vi "shooter_flywheel.vi"(8 "Low goal RPM":dbl=1500.0, 9 "High goal RPM":dbl=4000.0, 10 "Flywheel":bool, 11 "High goal?":bool) -> (2 "Flywheel RPM":cluster{"RPM":dbl, "Flywheel Setpoint RPM":dbl}(graph), 5 "error from goal":dbl, 7 "Closed-loop Error":dbl format="%.2f")   [LabVIEW 2020]
uses:
  <vilib>/Rock Robotics/WPI/ThirdParty/Phoenix-LabVIEW/Motor Controller/Controls/CTRE_Phoenix_MotorControl_ControlMode.ctl
  <vilib>/Rock Robotics/WPI/ThirdParty/JAS_Junk/TrajLib/SimpleMotorFF_Calculate.vi
  TitanLib/Lib/RPMToRawUnits-2048-CPR.vi
  <vilib>/Rock Robotics/WPI/ThirdParty/Phoenix-LabVIEW/Motor Controller/Get/CTRE_Phoenix_MotorController_GetSelectedSensorData.vi
  TitanLib/Lib/RawUnitsToRPM-2048-CPR.vi
  <vilib>/Rock Robotics/Network Tables/NT Write Number.vi
  <vilib>/Rock Robotics/WPI/ThirdParty/Phoenix-LabVIEW/Motor Controller/Get/CTRE_Phoenix_MotorController_GetVoltage.vi
  TitanLib/Lib/TitanLib.lvlib
  <vilib>/Rock Robotics/WPI/ThirdParty/JAS_Junk/TrajLib/Trajectory_Library.lvlib
panel:
  in  "Tolerance":dbl
  in  "kA":dbl
  out "Output Voltage":dbl(graph)
  in  "Flywheel PIDF":T1={"Set Constants"=FALSE, "P"=0.00029748, "I"=0.0, "D"=0.0, "F"=0.0, "I Zone"=0.0, "Cruise Velocity"=0, "Acceleration"=0, "Percent Deadband"=0.0}
  in  "kV":dbl=0.114
  in  "kS":dbl=0.1309
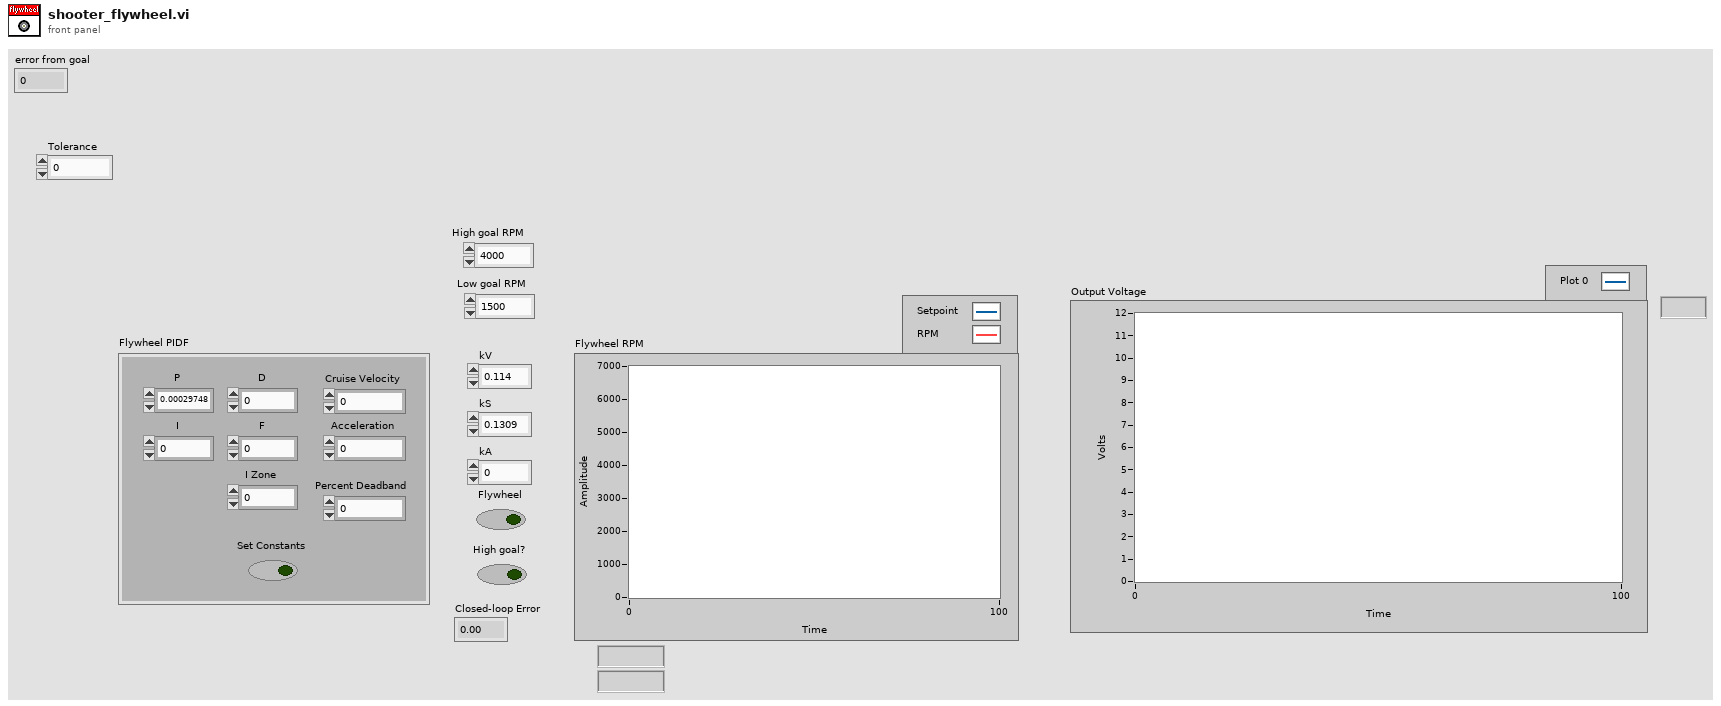
[diagram p1: front panel]
types:
  T1 = cluster{"Set Constants":bool, "P":dbl, "I":dbl, "D":dbl, "F":dbl, "I Zone":dbl, "Cruise Velocity":i32, "Acceleration":i32, "Percent Deadband":dbl}
  T2 = typedef "Trajectory_Library.lvlib/SIMPLE_MOTOR_FF.ctl" = cluster{"Ks":dbl, "Kv":dbl, "Ka":dbl}
  T3 = typedef "WPI_MotorControlDeviceRef.ctl" = cluster{"DeviceStatus":errorcluster, "Type":T4, "PWM":cluster{"PWM Channel":T5, "DeadBand":T6}, "CAN":cluster{"Device Number":u8, "SetOutput VI Ref":variant, "GetOutput VI Ref":variant, "Enable VI Ref":variant, "Disable VI Ref":variant, "Data":variant}, "Invert":bool, "DIO PWM":cluster{"PWM \"Enable\" Channel":T5, "DIOChannel":T7, "PWM Rate":dbl}}
  T4 = typedef "WPI_MotorControlType.ctl" = enum16{"PWM", "CAN", "DIO PWM"}
  T5 = typedef "FPGA_DIOPWMChannel.ctl" = enum8{"PWM 0", "PWM 1", "PWM 2", "PWM 3", "PWM 4", "PWM 5", "PWM 6", "PWM 7", "PWM 8", "PWM 9", "PWM MXP 0", "PWM MXP 1", "PWM MXP 2", "PWM MXP 3", "PWM MXP 4", "PWM MXP 5", "PWM MXP 6", "PWM MXP 7", "PWM MXP 8", "PWM MXP 9", "Invalid"}
  T6 = typedef "WPI_PWMDeadband.ctl" = cluster{"Name":string, "maxPositivePwm":i32, "minPositivePwm":i32, "centerPwm":i32, "maxNegativePwm":i32, "minNegativePwm":i32, "angularRange":u16}
  T7 = typedef "FPGA_DIOChannel.ctl" = enum8{"DIO 0", "DIO 1", "DIO 2", "DIO 3", "DIO 4", "DIO 5", "DIO 6", "DIO 7", "DIO 8", "DIO 9", "DIO MXP 0", "DIO MXP 1", "DIO MXP 2", "DIO MXP 3", "DIO MXP 4", "DIO MXP 5", "DIO MXP 6", "DIO MXP 7", "DIO MXP 8", "DIO MXP 9", "DIO MXP 10", "DIO MXP 11", "DIO MXP 12", "DIO MXP 13", "DIO MXP 14", "DIO MXP 15", "SPI Port CS1", "SPI Port CS2", "SPI Port CS3", "SPI Port MISO", "SPI Port MOSI", "Invalid"}
  T8 = typedef "CTRE_Phoenix_MotorControl_ControlMode.ctl" = u16
  T9 = enum16{"DemandType_Neutral", "DemandType_AuxPID", "DemandType_ArbitraryFeedForward"}
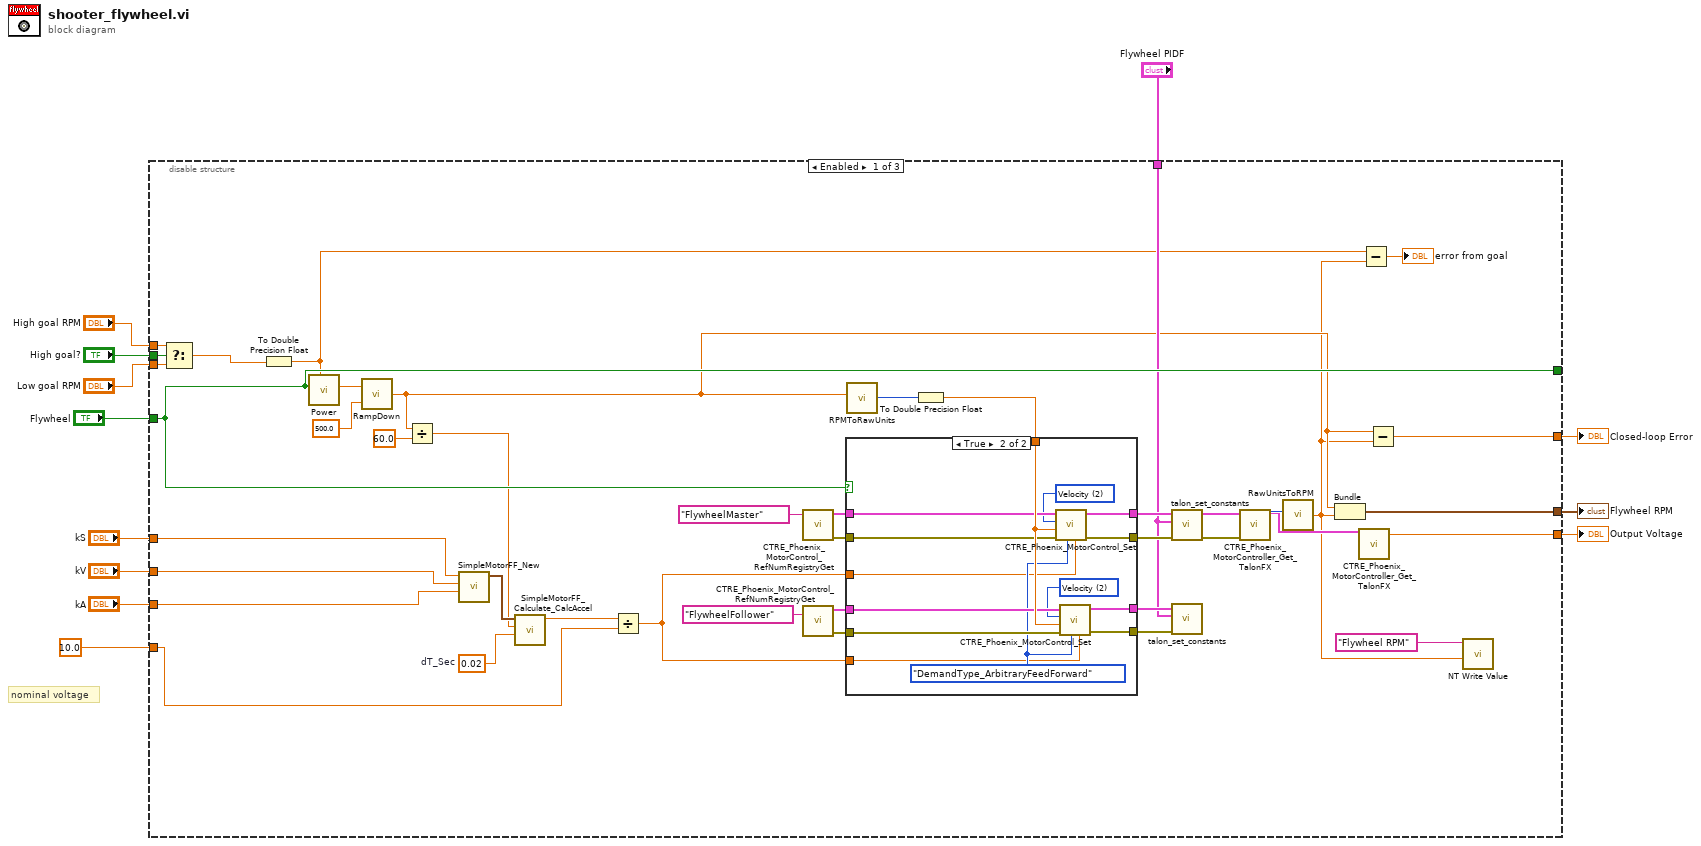
[diagram p0: block diagram]
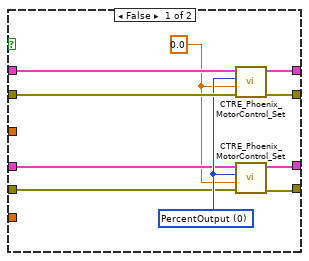
[diagram p2: hidden frame]
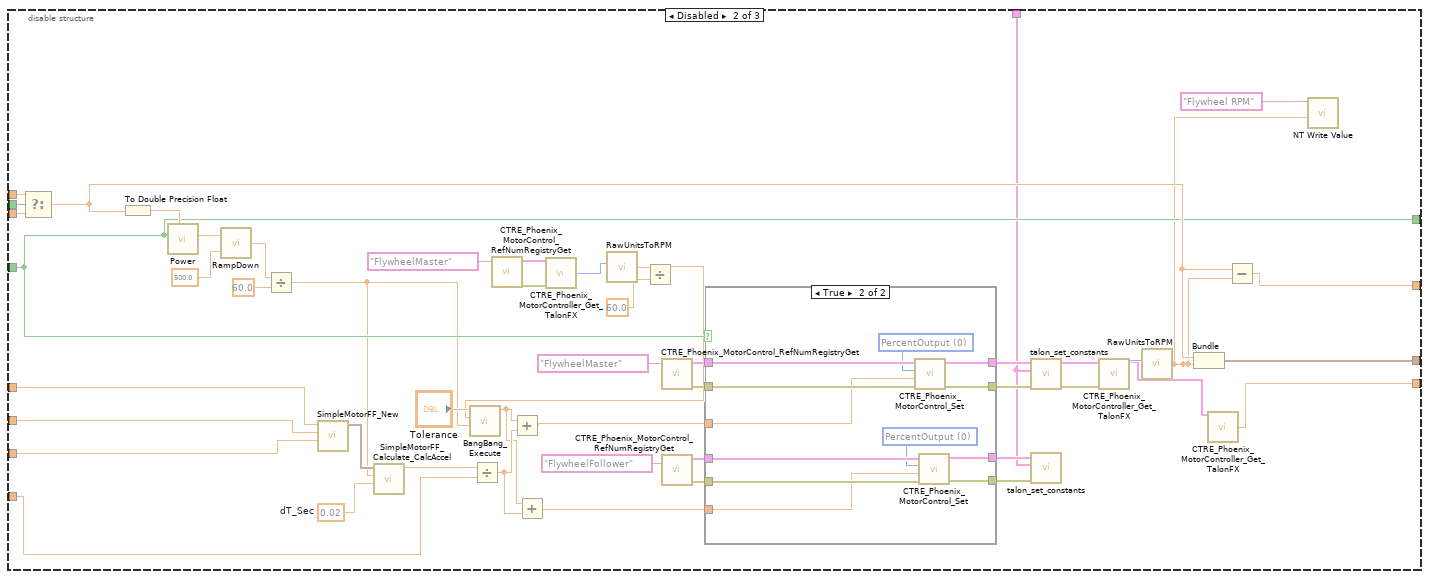
[diagram p3: hidden frame]
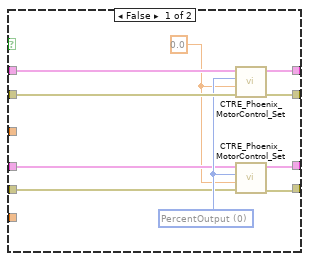
[diagram p4: hidden frame]
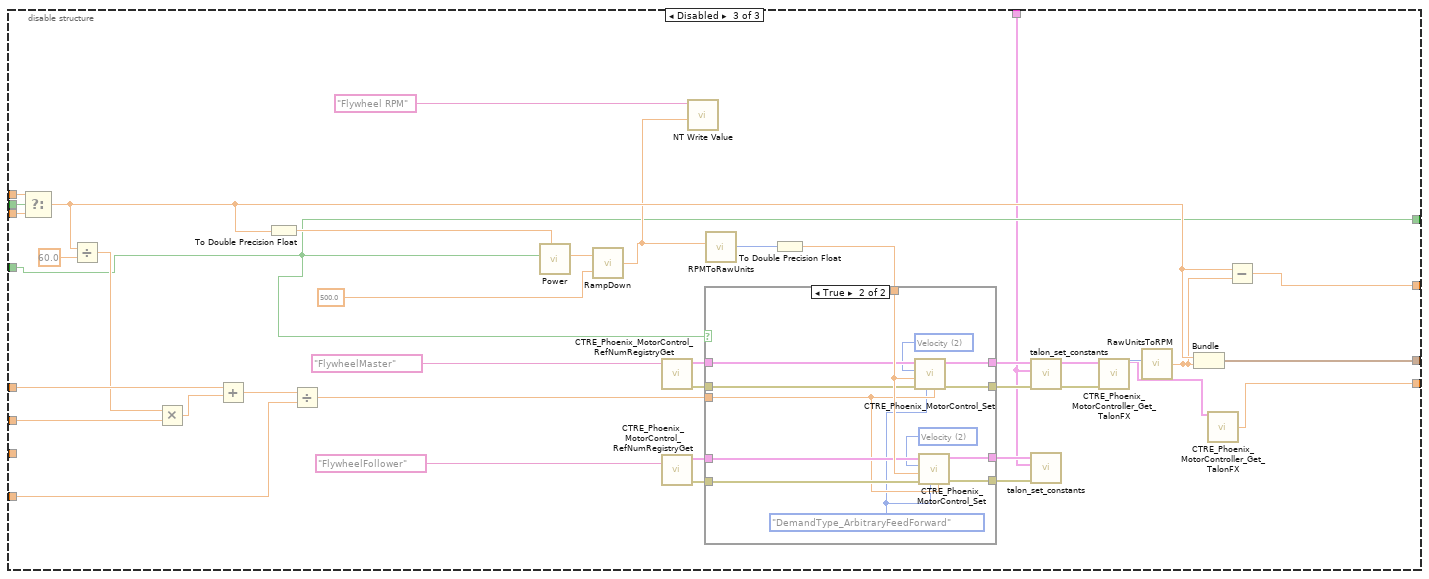
[diagram p5: hidden frame]
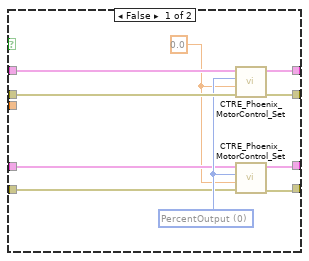
[diagram p6: hidden frame]
diagram:
  # "nominal voltage"
  n1 = disable-structure shown="Enabled" {
    disable-tunnel: 10.0 ("y") -> [w20 w94 w184]
    disable-tunnel: "kS" -> [w22 w95 w181]
    disable-tunnel: "kV" -> [w23 w96 w180]
    disable-tunnel: "High goal?" -> [w37 w112 w163]
    disable-tunnel: "Low goal RPM" -> [w36 w111 w162]
    disable-tunnel: "High goal RPM" -> [w35 w110 w161]
    disable-tunnel: [w34 w109 w160] -> w4
    disable-tunnel: [w31 w105 w154] -> _
    disable-tunnel: "Flywheel" -> [w31 w105 w154]
    disable-tunnel: "Flywheel PIDF" -> [w30 w104 w153]
    disable-tunnel: [w29 w103 w152] -> w3
    disable-tunnel: [w28 w102 w151] -> w2
    disable-tunnel: "kA" -> [w24 w97 _]
    frame Enabled {
      w26 = 0.02  # dT_Sec
      n2 = Select(t=w35, s=w37, f=w36) -> (s? t:f=w17:dbl)
      n3 = To Double Precision Float(number=w17) -> (double precision float=w15:dbl)
      n4 = call "Power.vi"("Positive Power"=w15, "Positive"=w31) -> ("Output"=w49:dbl)  [unwired: 9 in]
      n5 = call "RampDown.vi"("Decrease per Cycle"=500.0, "Input"=w49) -> ("Output"=w16:dbl)
      n6 = Divide(x=w16, y=60.0) -> (x/y=w21:dbl)
      n7 = call <vilib>:"SimpleMotorFF_New.vi"("Ka"=w24, "Kv"=w23, "Ks"=w22) -> ("SIMPLE_MOTOR_FF"=w25:T2)  [unwired: 8 in]
      n8 = call <vilib>:"SimpleMotorFF_Calculate_CalcAccel.vi"("dT_Sec"=w26, "Vel"=w21, "SIMPLE_MOTOR_FF"=w25) -> ("FeedForward"=w19:dbl)  [unwired: 8 in]
      n9 = Divide(x=w19, y=w20) -> (x/y=w18:dbl)
      n10 = call <vilib>:"CTRE_Phoenix_MotorControl_RefNumRegistryGet.vi"("refnum name"="FlywheelMaster") -> ("error out"=w46:errorcluster, "PhoenixMotorControlDevRef"=w45:T3)  [unwired: 9 in]
      n11 = call <vilib>:"CTRE_Phoenix_MotorControl_RefNumRegistryGet.vi"("refnum name"="FlywheelFollower") -> ("error out"=w48:errorcluster, "PhoenixMotorControlDevRef"=w47:T3)  [unwired: 9 in]
      n12 = call-poly "RPMToRawUnits.vi"("RPM"=w16) -> ("Raw Units"=w41:i32)  [unwired: 3 in]
      n13 = To Double Precision Float(number=w41) -> (double precision float=w40:dbl)
      n14 = case shown="True" w31 {
        tunnel: [w58 w78] -> w54
        tunnel: [w59 w77] -> w53
        tunnel: [w57 w76] -> w52
        tunnel: [w56 w75] -> w51
        tunnel: w40 -> [_ w74]
        tunnel: w48 -> [w60 w73]
        tunnel: w47 -> [w61 w72]
        tunnel: w46 -> [w64 w70]
        tunnel: w45 -> [w63 w69]
        tunnel: w18 -> [_ w66]
        tunnel: w18 -> [_ w65]
        frame False {
          w55 = 0.0 ("Output")
          w62 = T8 0 items=["PercentOutput"=0, "Position"=1, "Velocity"=2, "Current"=3, "Follower"=5, "MotionProfile"=6, "MotionMagic"=7, "MotionProfileArc"=10, "Disabled"=15] ("Control Mode")
          n15 = call <vilib>:"CTRE_Phoenix_MotorControl_Set.vi"("error in (no error)"=w64, "Output"=w55, "Control Mode"=w62, "PhoenixMotorControlDevRef"=w63) -> ("error out"=w57:errorcluster, "PhoenixMotorControlDevRef"=w56:T3)  [unwired: 6 in]
          n16 = call <vilib>:"CTRE_Phoenix_MotorControl_Set.vi"("error in (no error)"=w60, "Output"=w55, "Control Mode"=w62, "PhoenixMotorControlDevRef"=w61) -> ("error out"=w58:errorcluster, "PhoenixMotorControlDevRef"=w59:T3)  [unwired: 6 in]
        }
        frame True {
          w67 = T9."DemandType_ArbitraryFeedForward" ("DemandType")
          w71 = T8 2 items=["PercentOutput"=0, "Position"=1, "Velocity"=2, "Current"=3, "Follower"=5, "MotionProfile"=6, "MotionMagic"=7, "MotionProfileArc"=10, "Disabled"=15] ("Control Mode")
          w68 = T8 2 items=["PercentOutput"=0, "Position"=1, "Velocity"=2, "Current"=3, "Follower"=5, "MotionProfile"=6, "MotionMagic"=7, "MotionProfileArc"=10, "Disabled"=15] ("Control Mode")
          n17 = call <vilib>:"CTRE_Phoenix_MotorControl_Set.vi"("Demand1"=w65, "DemandType"=w67, "error in (no error)"=w70, "Output"=w74, "Control Mode"=w68, "PhoenixMotorControlDevRef"=w69) -> ("error out"=w76:errorcluster, "PhoenixMotorControlDevRef"=w75:T3)  [unwired: 4 in]
          n18 = call <vilib>:"CTRE_Phoenix_MotorControl_Set.vi"("Demand1"=w66, "DemandType"=w67, "error in (no error)"=w73, "Output"=w74, "Control Mode"=w71, "PhoenixMotorControlDevRef"=w72) -> ("error out"=w78:errorcluster, "PhoenixMotorControlDevRef"=w77:T3)  [unwired: 4 in]
        }
      }
      n19 = call "talon_set_constants.vi"("error in"=w52, "Constants"=w30, "PhoenixMotorControlDevRef"=w51) -> ("error out"=w38:errorcluster, "PhoenixMotorControlDevRef"=w39:T3)  [unwired: 7 in]
      n20 = call "talon_set_constants.vi"("error in"=w54, "Constants"=w30, "PhoenixMotorControlDevRef"=w53) -> ()  [unwired: 7 in, 2 out]
      n21 = call-poly <vilib>:"CTRE_Phoenix_MotorController_Get_TalonFX.vi"("PhoenixMotorControlDevRef"=w39, "error in"=w38) -> ("PhoenixMotorControlDevRef"=w33:T3, "Velocity (Raw Sensor Units per 100 ms)"=w42:i32)  [unwired: 10 in, 2 out]
      n22 = call-poly "RawUnitsToRPM.vi"("Raw Units"=w42) -> ("RPM"=w14:dbl)  [unwired: 3 in]
      n23 = Bundle("Output"=w16, "RPM"=w14) -> (w29:cluster{"Output":dbl, "RPM":dbl})  [unwired: 1 in]
      n24 = call-poly <vilib>:"CTRE_Phoenix_MotorController_Get_TalonFX.vi"("PhoenixMotorControlDevRef"=w33) -> ("Output Voltage"=w34:dbl)  [unwired: 10 in, 4 out]
      n25 = Subtract(x=w15, y=w14) -> (x-y=→"error from goal":dbl)
      n26 = Subtract(x=w16, y=w14) -> (x-y=w28:dbl)
      n27 = call-poly <vilib>:"NT Write Value.vi"("Numeric"=w14, "Name"="Flywheel RPM") -> ()  [unwired: 9 in, 1 out]
    }
    frame Disabled {
      w99 = 0.02  # dT_Sec
      n28 = Select(t=w110, s=w112, f=w111) -> (s? t:f=w107:dbl)
      n29 = To Double Precision Float(number=w107) -> (double precision float=w116:dbl)
      n30 = call "Power.vi"("Positive Power"=w116, "Positive"=w105) -> ("Output"=w123:dbl)  [unwired: 9 in]
      n31 = call "RampDown.vi"("Decrease per Cycle"=500.0, "Input"=w123) -> ("Output"=w101:dbl)
      n32 = Divide(x=w101, y=60.0) -> (x/y=w82:dbl)
      n33 = call <vilib>:"SimpleMotorFF_New.vi"("Ka"=w97, "Kv"=w96, "Ks"=w95) -> ("SIMPLE_MOTOR_FF"=w98:T2)  [unwired: 8 in]
      n34 = call <vilib>:"SimpleMotorFF_Calculate_CalcAccel.vi"("dT_Sec"=w99, "Vel"=w82, "SIMPLE_MOTOR_FF"=w98) -> ("FeedForward"=w93:dbl)  [unwired: 8 in]
      n35 = Divide(x=w93, y=w94) -> (x/y=w84:dbl)
      n36 = call <vilib>:"CTRE_Phoenix_MotorControl_RefNumRegistryGet.vi"("refnum name"="FlywheelMaster") -> ("error out"=w79:errorcluster, "PhoenixMotorControlDevRef"=w80:T3)  [unwired: 9 in]
      n37 = call-poly <vilib>:"CTRE_Phoenix_MotorController_Get_TalonFX.vi"("PhoenixMotorControlDevRef"=w80, "error in"=w79) -> ("Velocity (Raw Sensor Units per 100 ms)"=w86:i32)  [unwired: 10 in, 3 out]
      n38 = call-poly "RawUnitsToRPM.vi"("Raw Units"=w86) -> ("RPM"=w87:dbl)  [unwired: 3 in]
      n39 = Divide(x=w87, y=60.0) -> (x/y=w83:dbl)
      n40 = call <vilib>:"BangBang_Execute.vi"("Setpoint"=w82, "Measurment"=w83, "Tolerance"="Tolerance") -> ("ControlOutput"=w81:dbl)  [unwired: 6 in, 2 out]
      n41 = Add(x=w81, y=w84) -> (x+y=w91:dbl)
      n42 = Add(x=w81, y=w84) -> (x+y=w90:dbl)
      n43 = call <vilib>:"CTRE_Phoenix_MotorControl_RefNumRegistryGet.vi"("refnum name"="FlywheelMaster") -> ("error out"=w120:errorcluster, "PhoenixMotorControlDevRef"=w119:T3)  [unwired: 9 in]
      n44 = call <vilib>:"CTRE_Phoenix_MotorControl_RefNumRegistryGet.vi"("refnum name"="FlywheelFollower") -> ("error out"=w122:errorcluster, "PhoenixMotorControlDevRef"=w121:T3)  [unwired: 9 in]
      n45 = case shown="True" w105 {
        tunnel: [w132 w150] -> w128
        tunnel: [w133 w149] -> w127
        tunnel: [w131 w148] -> w126
        tunnel: [w130 w147] -> w125
        tunnel: w122 -> [w134 w146]
        tunnel: w121 -> [w135 w145]
        tunnel: w120 -> [w138 w143]
        tunnel: w119 -> [w137 w142]
        tunnel: w90 -> [_ w139]
        tunnel: w91 -> [_ w140]
        frame False {
          w129 = 0.0 ("Output")
          w136 = T8 0 items=["PercentOutput"=0, "Position"=1, "Velocity"=2, "Current"=3, "Follower"=5, "MotionProfile"=6, "MotionMagic"=7, "MotionProfileArc"=10, "Disabled"=15] ("Control Mode")
          n46 = call <vilib>:"CTRE_Phoenix_MotorControl_Set.vi"("error in (no error)"=w138, "Output"=w129, "Control Mode"=w136, "PhoenixMotorControlDevRef"=w137) -> ("error out"=w131:errorcluster, "PhoenixMotorControlDevRef"=w130:T3)  [unwired: 6 in]
          n47 = call <vilib>:"CTRE_Phoenix_MotorControl_Set.vi"("error in (no error)"=w134, "Output"=w129, "Control Mode"=w136, "PhoenixMotorControlDevRef"=w135) -> ("error out"=w132:errorcluster, "PhoenixMotorControlDevRef"=w133:T3)  [unwired: 6 in]
        }
        frame True {
          w144 = T8 0 items=["PercentOutput"=0, "Position"=1, "Velocity"=2, "Current"=3, "Follower"=5, "MotionProfile"=6, "MotionMagic"=7, "MotionProfileArc"=10, "Disabled"=15] ("Control Mode")
          w141 = T8 0 items=["PercentOutput"=0, "Position"=1, "Velocity"=2, "Current"=3, "Follower"=5, "MotionProfile"=6, "MotionMagic"=7, "MotionProfileArc"=10, "Disabled"=15] ("Control Mode")
          n48 = call <vilib>:"CTRE_Phoenix_MotorControl_Set.vi"("error in (no error)"=w143, "Output"=w140, "Control Mode"=w141, "PhoenixMotorControlDevRef"=w142) -> ("error out"=w148:errorcluster, "PhoenixMotorControlDevRef"=w147:T3)  [unwired: 6 in]
          n49 = call <vilib>:"CTRE_Phoenix_MotorControl_Set.vi"("error in (no error)"=w146, "Output"=w139, "Control Mode"=w144, "PhoenixMotorControlDevRef"=w145) -> ("error out"=w150:errorcluster, "PhoenixMotorControlDevRef"=w149:T3)  [unwired: 6 in]
        }
      }
      n50 = call "talon_set_constants.vi"("error in"=w126, "Constants"=w104, "PhoenixMotorControlDevRef"=w125) -> ("error out"=w113:errorcluster, "PhoenixMotorControlDevRef"=w114:T3)  [unwired: 7 in]
      n51 = call "talon_set_constants.vi"("error in"=w128, "Constants"=w104, "PhoenixMotorControlDevRef"=w127) -> ()  [unwired: 7 in, 2 out]
      n52 = call-poly <vilib>:"CTRE_Phoenix_MotorController_Get_TalonFX.vi"("PhoenixMotorControlDevRef"=w114, "error in"=w113) -> ("PhoenixMotorControlDevRef"=w108:T3, "Velocity (Raw Sensor Units per 100 ms)"=w115:i32)  [unwired: 10 in, 2 out]
      n53 = call-poly "RawUnitsToRPM.vi"("Raw Units"=w115) -> ("RPM"=w92:dbl)  [unwired: 3 in]
      n54 = Bundle("Low goal RPM"=w107, "RPM"=w92) -> (w103:cluster{"Low goal RPM":dbl, "RPM":dbl})  [unwired: 1 in]
      n55 = call-poly <vilib>:"CTRE_Phoenix_MotorController_Get_TalonFX.vi"("PhoenixMotorControlDevRef"=w108) -> ("Output Voltage"=w109:dbl)  [unwired: 10 in, 4 out]
      n56 = Subtract(x=w107, y=w92) -> (x-y=w102:dbl)
      n57 = call-poly <vilib>:"NT Write Value.vi"("Numeric"=w92, "Name"="Flywheel RPM") -> ()  [unwired: 9 in, 1 out]
    }
    frame Disabled {
      n58 = Select(t=w161, s=w163, f=w162) -> (s? t:f=w158:dbl)
      n59 = Divide(x=w158, y=60.0) -> (x/y=w169:dbl)
      n60 = Multiply(x=w169, y=w180) -> (x*y=w182:dbl)
      n61 = Add(x=w181, y=w182) -> (x+y=w183:dbl)
      n62 = To Double Precision Float(number=w158) -> (double precision float=w171:dbl)
      n63 = Divide(x=w183, y=w184) -> (x/y=w185:dbl)
      n64 = call "Power.vi"("Positive Power"=w171, "Positive"=w154) -> ("Output"=w178:dbl)  [unwired: 9 in]
      n65 = call "RampDown.vi"("Decrease per Cycle"=500.0, "Input"=w178) -> ("Output"=w155:dbl)
      n66 = call <vilib>:"CTRE_Phoenix_MotorControl_RefNumRegistryGet.vi"("refnum name"="FlywheelMaster") -> ("error out"=w175:errorcluster, "PhoenixMotorControlDevRef"=w174:T3)  [unwired: 9 in]
      n67 = call <vilib>:"CTRE_Phoenix_MotorControl_RefNumRegistryGet.vi"("refnum name"="FlywheelFollower") -> ("error out"=w177:errorcluster, "PhoenixMotorControlDevRef"=w176:T3)  [unwired: 9 in]
      n68 = call-poly <vilib>:"NT Write Value.vi"("Numeric"=w155, "Name"="Flywheel RPM") -> ()  [unwired: 9 in, 1 out]
      n69 = call-poly "RPMToRawUnits.vi"("RPM"=w155) -> ("Raw Units"=w167:i32)  [unwired: 3 in]
      n70 = To Double Precision Float(number=w167) -> (double precision float=w166:dbl)
      n71 = case shown="True" w154 {
        tunnel: [w193 w212] -> w189
        tunnel: [w194 w211] -> w188
        tunnel: [w192 w210] -> w187
        tunnel: [w191 w209] -> w186
        tunnel: w185 -> [_ w201]
        tunnel: w166 -> [_ w208]
        tunnel: w177 -> [w195 w207]
        tunnel: w176 -> [w196 w206]
        tunnel: w175 -> [w199 w204]
        tunnel: w174 -> [w198 w203]
        frame False {
          w190 = 0.0 ("Output")
          w197 = T8 0 items=["PercentOutput"=0, "Position"=1, "Velocity"=2, "Current"=3, "Follower"=5, "MotionProfile"=6, "MotionMagic"=7, "MotionProfileArc"=10, "Disabled"=15] ("Control Mode")
          n72 = call <vilib>:"CTRE_Phoenix_MotorControl_Set.vi"("error in (no error)"=w199, "Output"=w190, "Control Mode"=w197, "PhoenixMotorControlDevRef"=w198) -> ("error out"=w192:errorcluster, "PhoenixMotorControlDevRef"=w191:T3)  [unwired: 6 in]
          n73 = call <vilib>:"CTRE_Phoenix_MotorControl_Set.vi"("error in (no error)"=w195, "Output"=w190, "Control Mode"=w197, "PhoenixMotorControlDevRef"=w196) -> ("error out"=w193:errorcluster, "PhoenixMotorControlDevRef"=w194:T3)  [unwired: 6 in]
        }
        frame True {
          w200 = T9."DemandType_ArbitraryFeedForward" ("DemandType")
          w205 = T8 2 items=["PercentOutput"=0, "Position"=1, "Velocity"=2, "Current"=3, "Follower"=5, "MotionProfile"=6, "MotionMagic"=7, "MotionProfileArc"=10, "Disabled"=15] ("Control Mode")
          w202 = T8 2 items=["PercentOutput"=0, "Position"=1, "Velocity"=2, "Current"=3, "Follower"=5, "MotionProfile"=6, "MotionMagic"=7, "MotionProfileArc"=10, "Disabled"=15] ("Control Mode")
          n74 = call <vilib>:"CTRE_Phoenix_MotorControl_Set.vi"("Demand1"=w201, "DemandType"=w200, "error in (no error)"=w204, "Output"=w208, "Control Mode"=w202, "PhoenixMotorControlDevRef"=w203) -> ("error out"=w210:errorcluster, "PhoenixMotorControlDevRef"=w209:T3)  [unwired: 4 in]
          n75 = call <vilib>:"CTRE_Phoenix_MotorControl_Set.vi"("Demand1"=w201, "DemandType"=w200, "error in (no error)"=w207, "Output"=w208, "Control Mode"=w205, "PhoenixMotorControlDevRef"=w206) -> ("error out"=w212:errorcluster, "PhoenixMotorControlDevRef"=w211:T3)  [unwired: 4 in]
        }
      }
      n76 = call "talon_set_constants.vi"("error in"=w187, "Constants"=w153, "PhoenixMotorControlDevRef"=w186) -> ("error out"=w164:errorcluster, "PhoenixMotorControlDevRef"=w165:T3)  [unwired: 7 in]
      n77 = call "talon_set_constants.vi"("error in"=w189, "Constants"=w153, "PhoenixMotorControlDevRef"=w188) -> ()  [unwired: 7 in, 2 out]
      n78 = call-poly <vilib>:"CTRE_Phoenix_MotorController_Get_TalonFX.vi"("PhoenixMotorControlDevRef"=w165, "error in"=w164) -> ("PhoenixMotorControlDevRef"=w159:T3, "Velocity (Raw Sensor Units per 100 ms)"=w168:i32)  [unwired: 10 in, 2 out]
      n79 = call-poly "RawUnitsToRPM.vi"("Raw Units"=w168) -> ("RPM"=w157:dbl)  [unwired: 3 in]
      n80 = Bundle("Low goal RPM"=w158, "RPM"=w157) -> (w152:cluster{"Low goal RPM":dbl, "RPM":dbl})  [unwired: 1 in]
      n81 = call-poly <vilib>:"CTRE_Phoenix_MotorController_Get_TalonFX.vi"("PhoenixMotorControlDevRef"=w159) -> ("Output Voltage"=w160:dbl)  [unwired: 10 in, 4 out]
      n82 = Subtract(x=w158, y=w157) -> (x-y=w151:dbl)
    }
  }
  "Output Voltage" <- w4
  "Flywheel RPM" <- w3
  "Closed-loop Error" <- w2
